vi "Raycaster_CalcSpriteSize.vi"(9 "Inverse Matrix":fxp<+/-,32,16> format="%#_21g", 10 "Location Info":T1, 11 "Object Position":T4) -> (2 "Sprite Size":i16, 3 "Sprite X Position":i16)   [LabVIEW 2020]
uses:
  Controls/Map_Position.ctl
  Controls/Game_State.ctl
  Controls/Player_LocationInfo.ctl
  Controls/Player_LocationInfoAxis.ctl
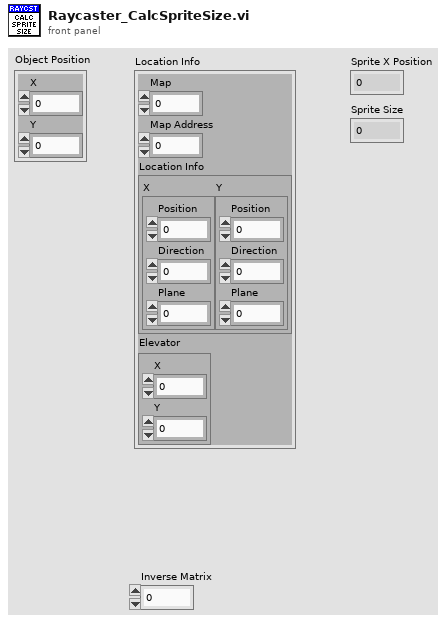
[diagram p1: front panel]
types:
  T1 = typedef "Game_State.ctl" = cluster{"Map":u8, "Map Address":u32, "Location Info":T2, "Elevator":T4}
  T2 = typedef "Player_LocationInfo.ctl" = cluster{"X":T3, "Y":T3}
  T3 = typedef "Player_LocationInfoAxis.ctl" = cluster{"Position":fxp<+/-,32,16>, "Direction":fxp<+/-,32,16>, "Plane":fxp<+/-,32,16>}
  T4 = typedef "Map_Position.ctl" = cluster{"X":fxp<+/-,32,16>, "Y":fxp<+/-,32,16>}
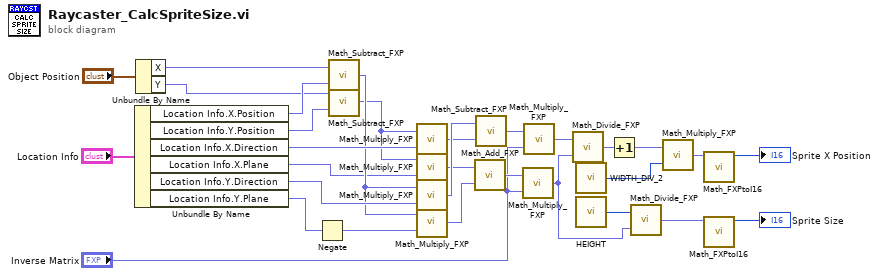
[diagram p0: block diagram]
diagram:
  n1 = Unbundle By Name("Location Info") -> ("Location Info.X.Position"=w30:fxp<+/-,32,16>, "Location Info.Y.Position"=w29:fxp<+/-,32,16>, "Location Info.X.Direction"=w27:fxp<+/-,32,16>, "Location Info.X.Plane"=w20:fxp<+/-,32,16>, "Location Info.Y.Direction"=w28:fxp<+/-,32,16>, "Location Info.Y.Plane"=w24:fxp<+/-,32,16>)
  n2 = Unbundle By Name("Object Position") -> ("X"=w6:fxp<+/-,32,16>, "Y"=w5:fxp<+/-,32,16>)
  n3 = Negate(x=w24) -> (-x=w22:fxp<+/-,33,17>)
  n4 = call "Math_Subtract_FXP.vi"("y"=w30, "x"=w6) -> ("x*y"=w23:fxp<+/-,32,16>)
  n5 = call "Math_Subtract_FXP.vi"("y"=w29, "x"=w5) -> ("x*y"=w21:fxp<+/-,32,16>)
  n6 = call "Math_Multiply_FXP.vi"("y"=w27, "x"=w21) -> ("x*y"=w25:fxp<+/-,32,16>)
  n7 = call "Math_Multiply_FXP.vi"("y"=w20, "x"=w21) -> ("x*y"=w18:fxp<+/-,32,16>)
  n8 = call "Math_Multiply_FXP.vi"("y"=w28, "x"=w23) -> ("x*y"=w26:fxp<+/-,32,16>)
  n9 = call "Math_Multiply_FXP.vi"("y"=w22, "x"=w23) -> ("x*y"=w17:fxp<+/-,32,16>)
  n10 = call "Math_Add_FXP.vi"("y"=w17, "x"=w18) -> ("x*y"=w16:fxp<+/-,32,16>)
  n11 = call "Math_Subtract_FXP.vi"("y"=w25, "x"=w26) -> ("x*y"=w19:fxp<+/-,32,16>)
  n12 = call "Math_Multiply_FXP.vi"("y"="Inverse Matrix", "x"=w16) -> ("x*y"=w8:fxp<+/-,32,16>)
  n13 = call "Math_Multiply_FXP.vi"("y"="Inverse Matrix", "x"=w19) -> ("x*y"=w15:fxp<+/-,32,16>)
  n14 = call "Math_Divide_FXP.vi"("y"=w8, "x"=w15) -> ("x*y"=w14:fxp<+/-,32,16>)
  n15 = call "WIDTH_DIV_2.vi"() -> ("WIDTH_DIV_2"=w12:i16)
  n16 = call "HEIGHT.vi"() -> ("HEIGHT"=w9:i16)
  n17 = Increment(x=w14) -> (x+1=w13:fxp<+/-,32,16>)
  n18 = call "Math_Divide_FXP.vi"("y"=w8, "x"=w9) -> ("x*y"=w10:fxp<+/-,32,16>)
  n19 = call "Math_Multiply_FXP.vi"("y"=w12, "x"=w13) -> ("x*y"=w11:fxp<+/-,32,16>)
  n20 = call "Math_FXPtoI16.vi"("FXP"=w11) -> ("I16"=→"Sprite X Position":i16)  [unwired: 10 in]
  n21 = call "Math_FXPtoI16.vi"("FXP"=w10) -> ("I16"=→"Sprite Size":i16)  [unwired: 10 in]
